vi "enum2str.vi"(1 "enum":variant) -> (0 "element":string)   [LabVIEW 2015]
uses:
  <vilib>/Utility/Data Type/NI_Data Type.lvlib
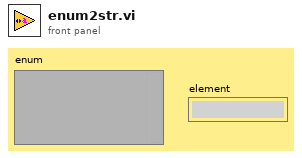
[diagram p1: front panel]
types:
  T1 = typedef "NI_Data Type.lvlib/Data Type.ctl" = enum8{"Invalid Type", "Void", "I8", "I16", "I32", "I64", "U8", "U16", "U32", "U64", "Single Float", "Double Float", "Extended Float", "Single Complex", "Double Complex", "Extended Complex", "Enum U8", "Enum U16", "Enum U32", "Enum U64", "Single Float With Unit", "Double Float With Unit", "Extended Float With Unit", "Single Complex with Unit", "Double Complex with Unit", "Extended Complex with Unit", "Boolean", "String", "Path", "Picture", "Tag", "Array", "Cluster", "Variant", "LV Variant", "Waveform", "Timestamp", "Digital Waveform", "Digital Data", "ExpressData", "Refnum", "External Data", "VI", "Poly VI", "LabVIEW Class Instance", "Fixed Point"}
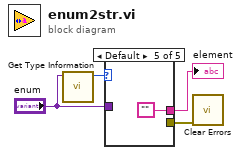
[diagram p0: block diagram]
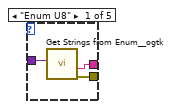
[diagram p2: hidden frame]
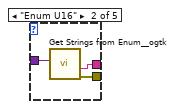
[diagram p3: hidden frame]
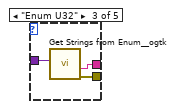
[diagram p4: hidden frame]
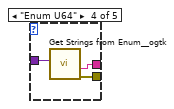
[diagram p5: hidden frame]
diagram:
  n1 = call <vilib>:"Get Type Information.vi"("Variant"="enum") -> ("Type"=w4:T1)  [unwired: 6 in, 4 out]
  n2 = case shown="Default" w4 {
    tunnel: [w6 w9 w12 w15 ""] -> w3
    tunnel: "enum" -> [w7 w10 w13 w16 _]
    tunnel: [w5 w8 w11 w14 _] -> w1
    frame "Enum U8" {
      n3 = call <userlib>:"Get Strings from Enum__ogtk.vi"("Enum"=w7) -> ("error out"=w5:errorcluster, "String Value"=w6:string)  [unwired: 7 in, 2 out]
    }
    frame "Enum U16" {
      n4 = call <userlib>:"Get Strings from Enum__ogtk.vi"("Enum"=w10) -> ("error out"=w8:errorcluster, "String Value"=w9:string)  [unwired: 7 in, 2 out]
    }
    frame "Enum U32" {
      n5 = call <userlib>:"Get Strings from Enum__ogtk.vi"("Enum"=w13) -> ("error out"=w11:errorcluster, "String Value"=w12:string)  [unwired: 7 in, 2 out]
    }
    frame "Enum U64" {
      n6 = call <userlib>:"Get Strings from Enum__ogtk.vi"("Enum"=w16) -> ("error out"=w14:errorcluster, "String Value"=w15:string)  [unwired: 7 in, 2 out]
    }
    frame Default {
    }
  }
  "element" <- w3
  n7 = call <vilib>:"Clear Errors.vi"("error in (no error)"=w1) -> ()  [unwired: 5 in, 2 out]
